vi "SetDigitalOutput.vi"(5 "value":i32, 6 "return immediately":bool, 7 "word":i32 min=0 max=2 step=1, 8 "error in (no error)":errorcluster, 9 "taskId":i32(ring) items=["TLibrary", "T01", "T02", "T03", "T04", "T05", "T06", "T07", "T08", "T09", "T10", "T11", "T12", "T13", "T14", "T15", "T16", "T17", "T18", "T19", "T20", "T21", "T22", "T23", "T24", "T25", "T26", "T27", "T28", "T29", "T30", "T31"], 10 "axis name":string, 11 "controller in":refnum<k24>) -> (0 "error out":errorcluster, 3 "controller out":refnum<k24>)   [LabVIEW 2010]
uses:
  c:/aerotech/controller/stable/a3200/pc/labview/2010/bin/Aerotech.A3200.dll
  bin/Aerotech.A3200.dll
  c:/aerotech/controller/stable/a3200/pc/labview/2010/bin/Aerotech.A3200.LabVIEW.dll
  bin/Aerotech.A3200.LabVIEW.dll
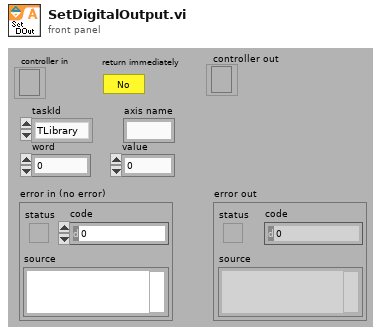
[diagram p1: front panel]
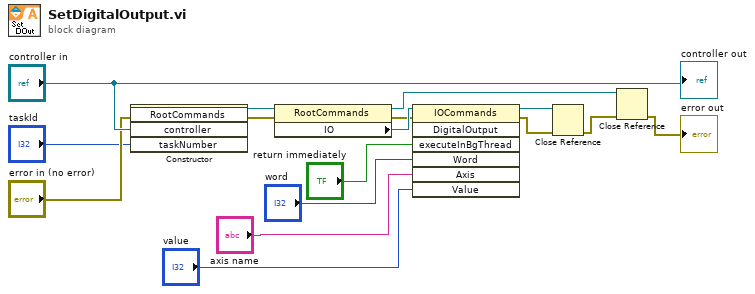
[diagram p0: block diagram]
diagram:
  n1 = constructor class="RootCommands"(error in="error in (no error)", "controller"="controller in", "taskNumber"="taskId") -> (reference out=w14:refnum<k24>, error out=w13:errorcluster)  [unwired: 2 in, 3 out]
  n2 = property class="RootCommands"(reference=w14, error in=w13) -> (reference out=w9:refnum<k24>, error out=w8:errorcluster, "IO"=w12:refnum<k24>)
  n3 = invoke class="IOCommands" method="DigitalOutput"(reference=w12, error in=w8, "executeInBgThread"="return immediately", "Word"="word", "Axis"="axis name", "Value"="value") -> (reference out=w11:refnum<k24>, error out=w10:errorcluster)  [unwired: 1 in, 5 out]
  n4 = Close Reference(reference=w11, error in (no error)=w10) -> (error out=w16:errorcluster)
  n5 = Close Reference(reference=w9, error in (no error)=w16) -> (error out=→"error out":errorcluster)
  "controller out" <- "controller in"
